vi "küvözler için nem ölçüm sistemi ve mail ile geri bildirim.vi"() -> ()   [LabVIEW 2017]
uses:
  <vilib>/Instr/_visa.llb/VISA Configure Serial Port (Instr).vi
panel:
  out "Gönderilen":bool=TRUE
  out "sıcaklık":string
  out "nem":string
  in  "Mail gönderim günü":timestamp
  out "Gerçek Zaman":timestamp
  out "nem":i32(knob) scale=0.0..100.0
  out "sıcaklık":i32(slide) scale=0.0..100.0
  out "nem":i32
  in  "stop":bool
  out "sıcaklık":i32
  in  "Serial Port":refnum<visa-resource-name>
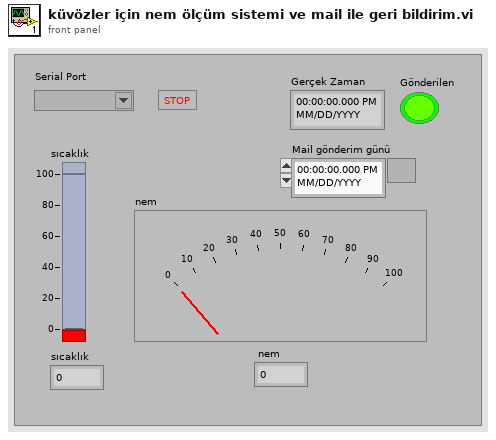
[diagram p1: front panel]
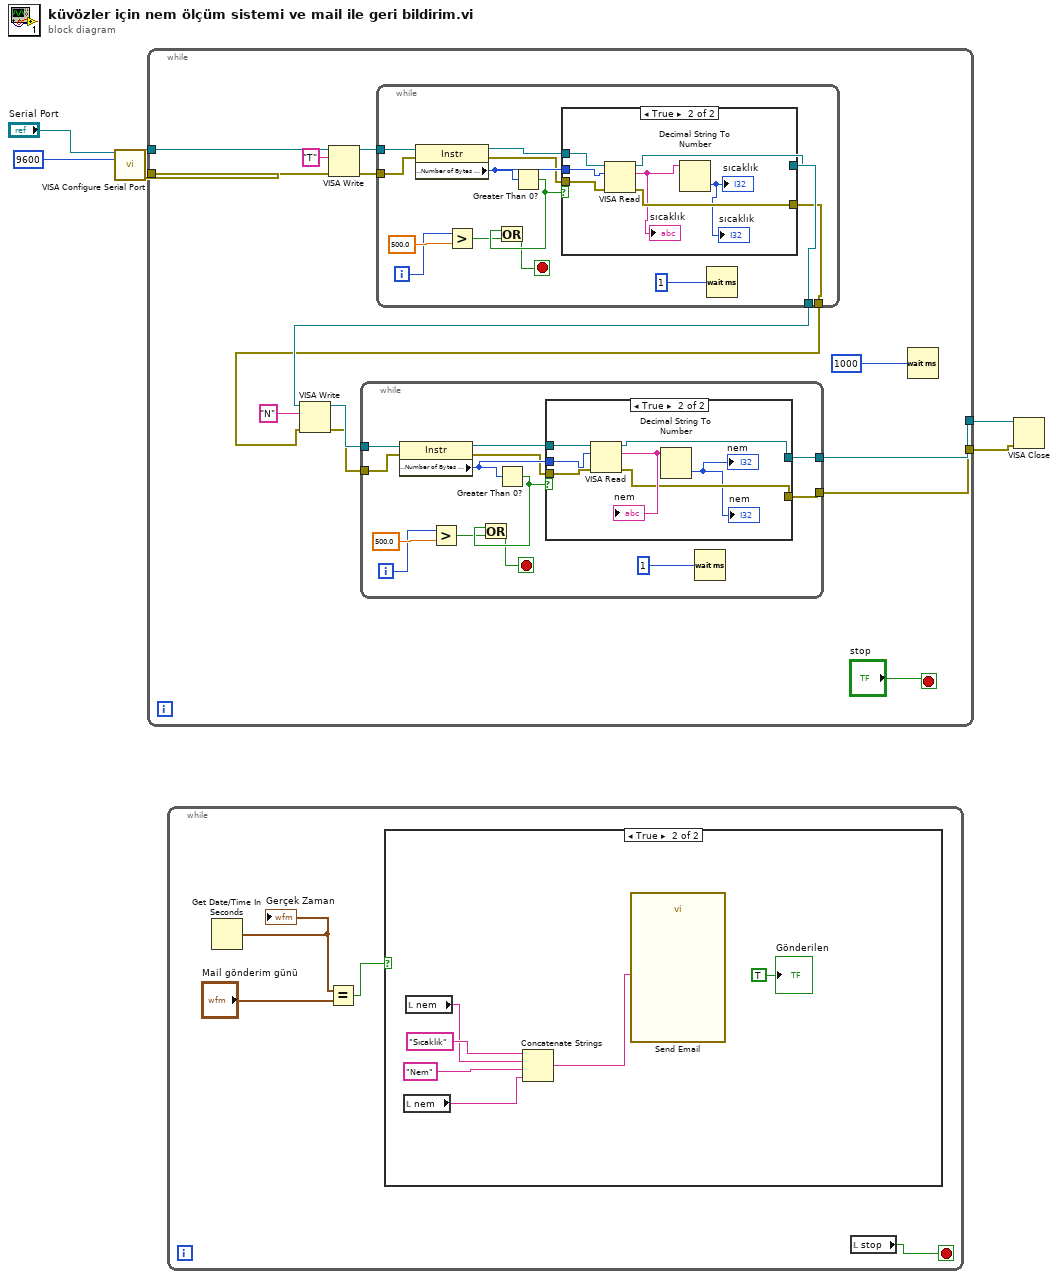
[diagram p0: block diagram]
diagram:
  n1 = call-poly "VISA Configure Serial Port"("VISA resource name"="Serial Port", "baud rate (9600)"=u32 9600) -> ("VISA resource name out"=w4:refnum<visa-resource-name>, "error out"=w3:errorcluster)  [unwired: 12 in]
  n2 = while {
    tunnel: w4 -> [w20]
    tunnel: w3 -> [w19]
    tunnel: [w8] -> w2
    tunnel: [w7] -> w1
    stop <- "stop" stop-if-true
    n3 = VISA Write(VISA resource name=w20, write buffer="T", error in (no error)=w19) -> (VISA resource name out=w17:refnum<visa-resource-name>, error out=w16:errorcluster)  [unwired: 1 out]
    n4 = while {
      tunnel: w17 -> [w55]
      tunnel: w16 -> [w54]
      tunnel: [w44] -> w10
      tunnel: [w43] -> w9
      i -> [w48]
      stop <- w45 stop-if-true
      n5 = property class="Instr"(reference=w55, error in=w54) -> (reference out=w53:refnum<visa-resource-name>, error out=w51:errorcluster, "Serial Settings:Number of Bytes at Serial Port"=w52:u32)
      n6 = Greater?(x=w48, y=500.0) -> (0:w46:bool)
      n7 = Greater Than 0?(x=w52) -> (x > 0?=w47:bool)
      n8 = Or(x=w47, y=w46) -> (x .or. y?=w45:bool)
      n9 = case shown="True" w47 {
        tunnel: w53 -> [w57 w64]
        tunnel: w52 -> [_ w63]
        tunnel: w51 -> [w56 w62]
        tunnel: [w57 w61] -> w44
        tunnel: [w56 w60] -> w43
        frame False {
        }
        frame True {
          n10 = VISA Read(VISA resource name=w64, byte count=w63, error in (no error)=w62) -> (VISA resource name out=w61:refnum<visa-resource-name>, read buffer=w58:string, error out=w60:errorcluster)  [unwired: 1 out]
          "sıcaklık" <- w58
          n11 = Decimal String To Number(string=w58) -> (number=→"sıcaklık" →"sıcaklık":i32)  [unwired: 2 in, 1 out]
        }
      }
      n12 = Wait (ms)(milliseconds to wait=u32 1) -> ()  [unwired: 1 out]
    }
    n13 = VISA Write(VISA resource name=w10, write buffer="N", error in (no error)=w9) -> (VISA resource name out=w12:refnum<visa-resource-name>, error out=w11:errorcluster)  [unwired: 1 out]
    n14 = while {
      tunnel: w12 -> [w33]
      tunnel: w11 -> [w32]
      tunnel: [w28] -> w8
      tunnel: [w27] -> w7
      i -> [w24]
      stop <- w21 stop-if-true
      n15 = property class="Instr"(reference=w33, error in=w32) -> (reference out=w31:refnum<visa-resource-name>, error out=w29:errorcluster, "Serial Settings:Number of Bytes at Serial Port"=w30:u32)
      n16 = Greater?(x=w24, y=500.0) -> (0:w22:bool)
      n17 = Greater Than 0?(x=w30) -> (x > 0?=w23:bool)
      n18 = Or(x=w23, y=w22) -> (x .or. y?=w21:bool)
      n19 = case shown="True" w23 {
        tunnel: w31 -> [w35 w42]
        tunnel: w30 -> [_ w41]
        tunnel: w29 -> [w34 w40]
        tunnel: [w35 w38] -> w28
        tunnel: [w34 w37] -> w27
        frame False {
        }
        frame True {
          n20 = VISA Read(VISA resource name=w42, byte count=w41, error in (no error)=w40) -> (VISA resource name out=w38:refnum<visa-resource-name>, read buffer=w39:string, error out=w37:errorcluster)  [unwired: 1 out]
          "nem" <- w39
          n21 = Decimal String To Number(string=w39) -> (number=→"nem" →"nem":i32)  [unwired: 2 in, 1 out]
        }
      }
      n22 = Wait (ms)(milliseconds to wait=u32 1) -> ()  [unwired: 1 out]
    }
    n23 = Wait (ms)(milliseconds to wait=u32 1000) -> ()  [unwired: 1 out]
  }
  n24 = while {
    stop <- w65 stop-if-true
    n25 = Get Date/Time In Seconds() -> (seconds since 1Jan1904=w68:timestamp)
    "Gerçek Zaman" <- w68
    n26 = Equal?(x=w68, y="Mail gönderim günü") -> (x = y?=w66:bool)
    n27 = case shown="True" w66 {
      frame False {
      }
      frame True {
        n28 = local read "nem"() -> (w72:string)
        n29 = local read "nem"() -> (w71:string)
        n30 = Concatenate Strings("Sıcaklık" ("string"), w71, "Nem" ("string"), w72) -> (w70:string)
        n31 = call "Send Email"("Message"=w70) -> ()  [unwired: 10 in, 1 out]
        "Gönderilen" <- TRUE
      }
    }
    n32 = local read "stop"() -> (w65:bool)
  }
  n33 = VISA Close(VISA resource name=w2, error in (no error)=w1) -> ()  [unwired: 1 out]
